vi "Data Available Queue.vi"(11 "error in (no error)":errorcluster) -> (6 "Waveform Graph":dbl[][](graph), 8 "Abort Send Data Queue":bool, 10 "AI Waveforms":dbl[][](array[numeric]), 14 "Timed out":bool, 15 "error out":errorcluster)   [LabVIEW 2020]
uses:
  DAQ Engine VIs/PXI Globals.vi
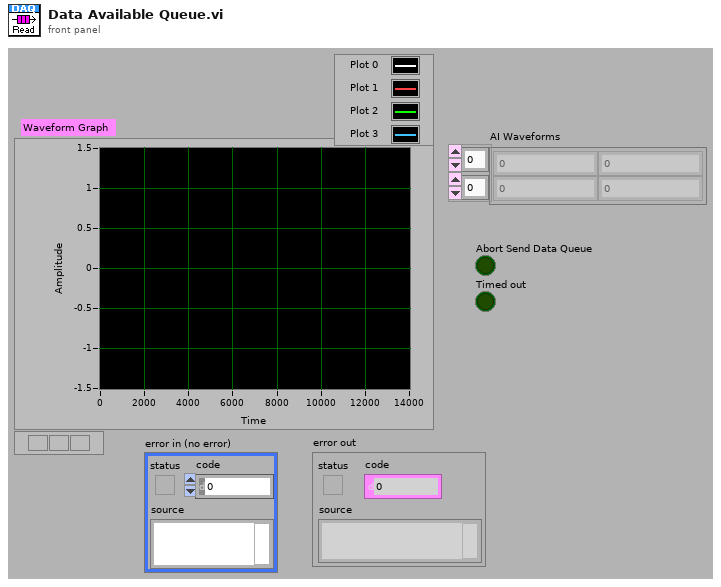
[diagram p1: front panel]
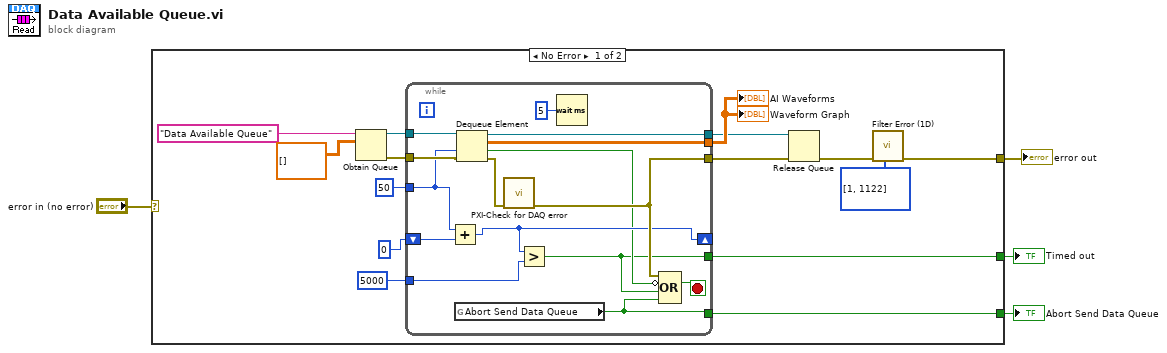
[diagram p0: block diagram]
diagram:
  n1 = case shown="No Error" "error in (no error)" {
    selector: "error in (no error)" -> [_ w35]
    tunnel: [w10 w35] -> w4
    tunnel: [w6 _] -> w2
    tunnel: [w5 _] -> w1
    frame No Error {
      n2 = Obtain Queue(name (unnamed)="Data Available Queue", element data type=dbl[][] [] ("AI Waveforms 2")) -> (queue out=w17:refnum<queue>, error out=w14:errorcluster)  [unwired: 3 in, 1 out]
      n3 = while {
        tunnel: [w27] -> w12
        tunnel: w17 -> [w34]
        tunnel: [w33] -> w16
        tunnel: [w32] -> w15
        tunnel: w14 -> [w29]
        tunnel: 50 ("timeout in ms (-1)") -> [w25]
        shift-right: [w24] -> _
        shift-left: 0 -> [w26]
        tunnel: 5000 ("timeout in ms (-1)") -> [w23]
        tunnel: [w21] -> w6
        tunnel: [w20] -> w5
        stop <- w31 stop-if-true
        n4 = Add(x=w25, y=w26) -> (x+y=w24:i32)
        n5 = global read "PXI Globals.vi" "Abort Send Data Queue"() -> (w21:bool)
        n6 = Dequeue Element(queue=w34, timeout in ms (-1)=w25, error in (no error)=w29) -> (queue out=w32:refnum<queue>, element=w33:dbl[][], timed out?=w22:bool, error out=w30:errorcluster)
        n7 = call "PXI-Check for DAQ error.vi"("error in (no error)"=w30) -> ("error out"=w27:errorcluster)  [unwired: 14 in]
        n8 = Greater?(x=w24, y=w23) -> (0:w20:bool)
        n9 = Wait (ms)(milliseconds to wait=u32 5) -> ()  [unwired: 1 out]
        n10 = Compound Arithmetic op=OR(w27, invert w22, w20, w21) -> (w31:bool)
      }
      "AI Waveforms" <- w16
      "Waveform Graph" <- w16
      n11 = Release Queue(queue=w15, error in (no error)=w12) -> (error out=w11:errorcluster)  [unwired: 1 in, 2 out]
      n12 = call "Filter Error (1D).vi"("error in (no error)"=w11, "Array"=i32[] [1, 1122]) -> ("error out"=w10:errorcluster)  [unwired: 9 in]
    }
    frame Error {
    }
  }
  "error out" <- w4
  "Abort Send Data Queue" <- w2
  "Timed out" <- w1
